vi "Find Slope and Intercept.vi"() -> ()   [LabVIEW 2020]
uses:
  Control/State - eFGV.ctl
  <vilib>/Analysis/NI_AALPro.lvlib
  <vilib>/Analysis/6fits.llb/Curve Fitting Criteria.ctl
  <vilib>/DAQmx/create/channels.llb/DAQmx Create Channel (AI-Pressure-Bridge-Table).vi
panel:
  in  "Delete index (row)":i32
  in  "Delete":bool
  out "intercept":dbl=-0.0
  out "slope":dbl=1000.0
  in  "Insert":bool
  in  "Readings":dbl[][](array[numeric])=[[0.0315564, 0.0], [0.22232425212860107, 573.0], [0.36340194940567017, 994.0], [0.7131384611129761, 2041.0], [1.0534383058547974, 3060.0], [1.3849239349365234, 4052.0], [1.7391854524612427, 5112.0], [2.0930733680725098, 6170.0], [2.4199507236480713, 7148.0], [2.762993812561035, 8174.0], [3.096597909927368, 9172.0], [3.4271647930145264, 10161.0], [3.730435609817505, 11067.0], [4.083857536315918, 12126.0], [4.432881832122803, 13172.0], [4.811169147491455, 14314.0], [5.0111083984375, 15151.0], [5.050300121307373, 16137.0], [5.08100700378418, 17097.0], [5.111919403076172, 18072.0], [5.147753715515137, 19172.0], [5.178903102874756, 20156.0], [5.262630939483643, 22859.0], [5.2826104164123535, 23500.0]]
  out "Sensor Reading (AI0)":sgl=0.63656884
  in  "Real Pressure":dbl
  in  "stop":bool
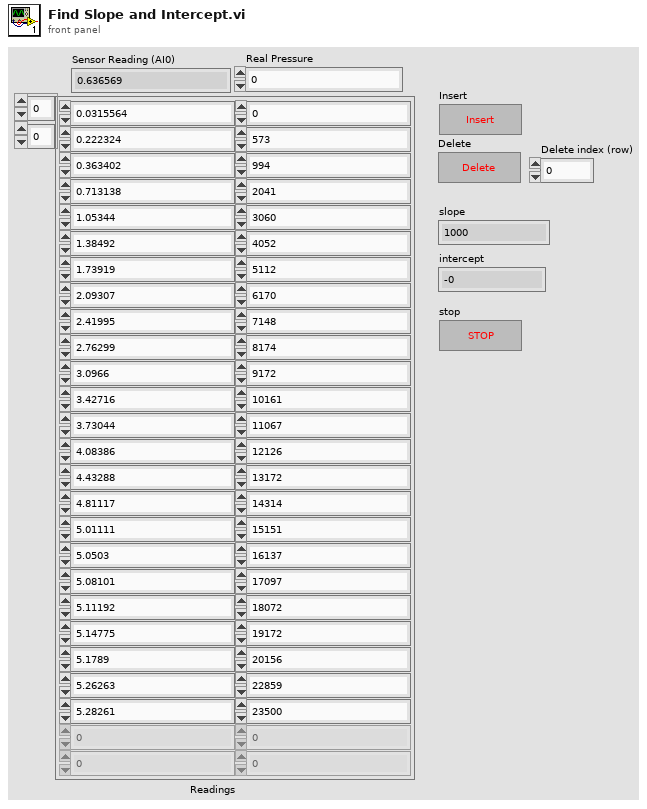
[diagram p1: front panel]
types:
  T1 = typedef "State - eFGV.ctl" = enum16{"Init", "Read", "Write", "Exit"}
  T2 = typedef "NI_AALPro.lvlib/Curve Fitting Criteria.ctl" = u16
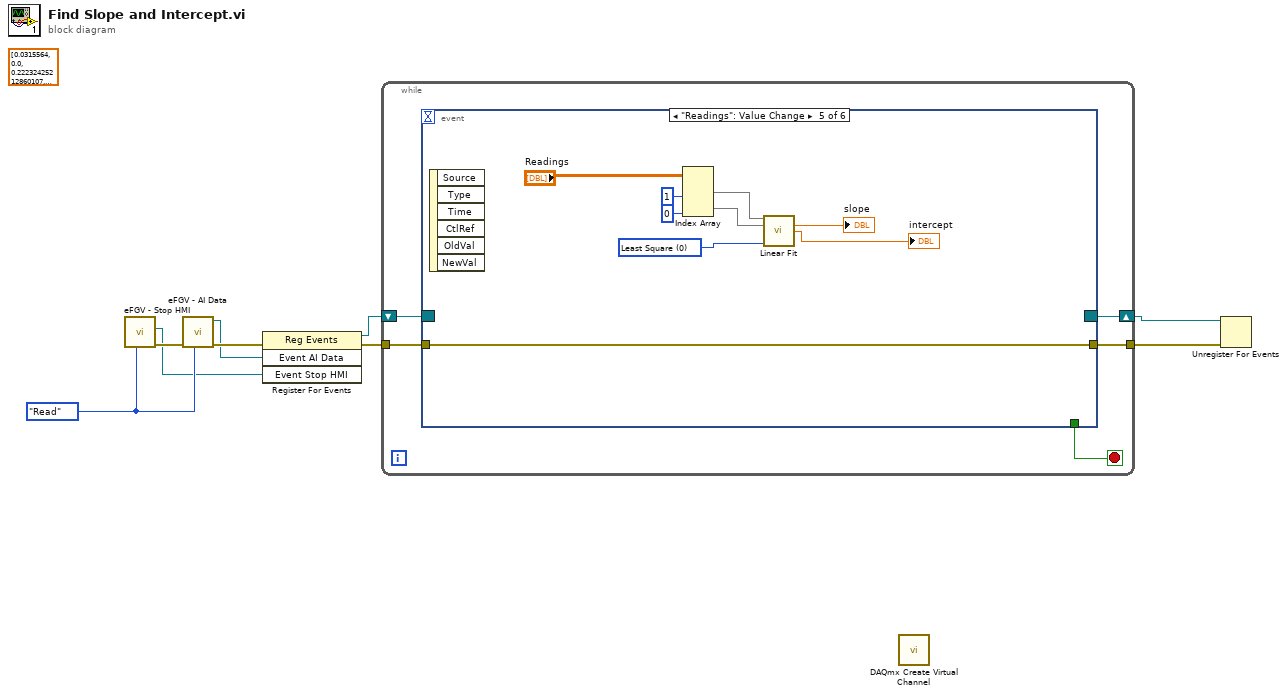
[diagram p0: block diagram]
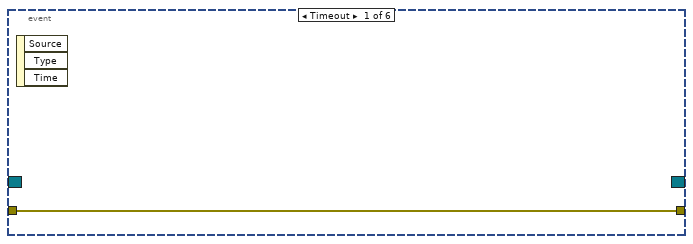
[diagram p2: hidden frame]
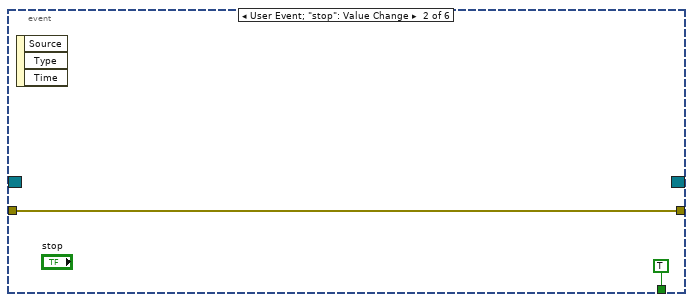
[diagram p3: hidden frame]
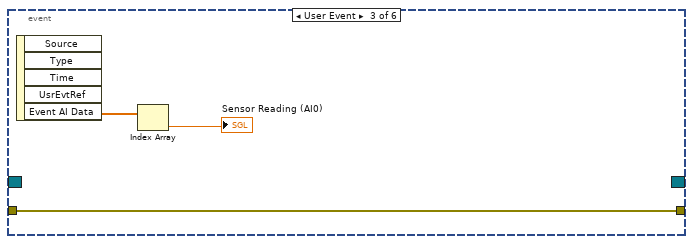
[diagram p4: hidden frame]
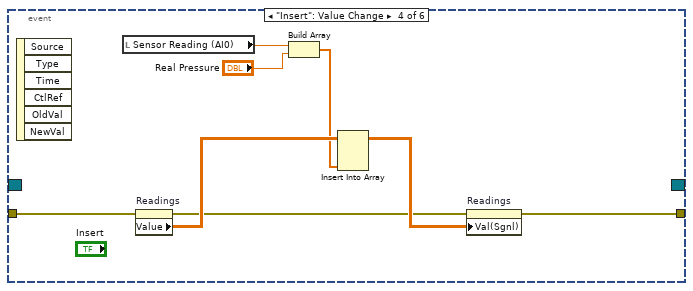
[diagram p5: hidden frame]
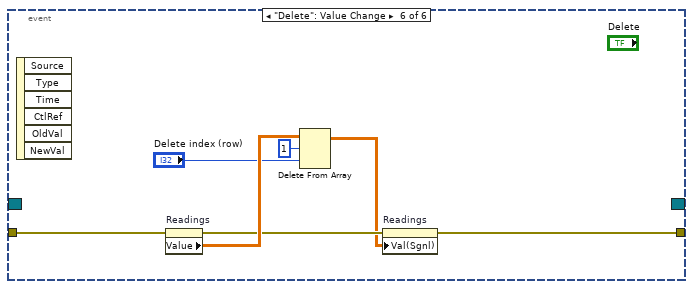
[diagram p6: hidden frame]
diagram:
  (unwired) dbl[][] [[0.0315564, 0.0], [0.22232425212860107, 573.0], [0.36340194940567017, 994.0], [0.7131384611129761, 2041.0], [1.0534383058547974, 3060.0], [1.3849239349365234, 4052.0], [1.7391854524612427, 5112.0], [2.0930733680725098, 6170.0], [2.4199507236480713, 7148.0], [2.762993812561035, 8174.0], [3.096597909927368, 9172.0], [3.4271647930145264, 10161.0], [3.730435609817505, 11067.0], [4.083857536315918, 12126.0], [4.432881832122803, 13172.0], [4.811169147491455, 14314.0], [5.0111083984375, 15151.0], [5.050300121307373, 16137.0], [5.08100700378418, 17097.0], [5.111919403076172, 18072.0], [5.147753715515137, 19172.0], [5.178903102874756, 20156.0], [5.262630939483643, 22859.0], [5.2826104164123535, 23500.0]] ("Readings")
  w4 = State_-_eFGV."Read" ("States")
  n1 = call "eFGV - Stop HMI.vi"("Action"=w4) -> ("Error Out"=w5:errorcluster, "Event Stop HMI"=w3:refnum<user-event>)  [unwired: 8 in, 1 out]
  n2 = call "eFGV - AI Data.vi"("States"=w4, "Error In"=w5) -> ("Error Out"=w9:errorcluster, "Event AI Data"=w6:refnum<user-event>)  [unwired: 8 in]
  n3 = register-events(error in=w9, w6, w3) -> (reference out=w7:refnum<event-registration>, error out=w8:errorcluster)  [unwired: 1 in]
  n4 = while {
    tunnel: w8 -> [w14]
    shift-right: [w12] -> w1
    shift-left: w7 -> [w13]
    tunnel: [w11] -> w2
    stop <- w10 stop-if-true
    n5 = event shown="[4] \"Readings\": Value Change" {
      selector: w13 -> [_ _ _ _ _ _]
      dyn-events: [_ _ _ _ _ _] -> w12
      timeout: _ -> [_ _ _ _ _ _]
      tunnel: w14 -> [w15 w17 w18 w28 w29 w44]
      tunnel: [w15 w17 w18 w25 w29 w38] -> w11
      tunnel: [_ TRUE _ _ _ _] -> w10
      event Timeout {
        n6 = event-data() -> ()  [unwired: 1 in, 3 out]
      }
      event User Event; "stop": Value Change {
        n7 = event-data() -> ()  [unwired: 1 in, 3 out]
      }
      event User Event {
        n8 = event-data() -> ("Event AI Data"=w20:sgl[])  [unwired: 1 in, 4 out]
        n9 = Index Array(array=w20) -> (element=→"Sensor Reading (AI0)":sgl)  [unwired: 1 in]
      }
      event "Insert": Value Change {
        n10 = event-data() -> ()  [unwired: 1 in, 6 out]
        n11 = local read "Sensor Reading (AI0)"() -> (w23:sgl)
        n12 = property on="Readings" class="Arr (strict)"(error in=w28) -> (error out=w24:errorcluster, "Value"=w27:dbl[][])  [unwired: 1 in, 1 out]
        n13 = Build Array(w23, "Real Pressure") -> (w21:dbl[])
        n14 = Insert Into Array(array=w27, new element=w21) -> (w26:dbl[][])  [unwired: 2 in]
        n15 = property on="Readings" class="Arr (strict)"(error in=w24, "Val(Sgnl)"=w26) -> (error out=w25:errorcluster)  [unwired: 1 in, 1 out]
      }
      event "Readings": Value Change {
        w37 = T2 0 items=["Least Square", "Least Absolute Residual", "Bisquare"] ("method")
        n16 = event-data() -> ()  [unwired: 1 in, 6 out]
        n17 = Index Array(array="Readings", index (col) #1=1 ("disabled index (col)"), index (col) #2=0 ("index (col)")) -> (element #1=w33:dbl[], element #2=w32:dbl[])  [unwired: 2 in]
        n18 = call <vilib>:"Linear Fit.vi"("Y"=w33, "X"=w32, "method"=w37) -> ("slope"=→"slope":dbl, "intercept"=→"intercept":dbl)  [unwired: 8 in, 3 out]
      }
      event "Delete": Value Change {
        n19 = event-data() -> ()  [unwired: 1 in, 6 out]
        n20 = property on="Readings" class="Arr (strict)"(error in=w44) -> (error out=w40:errorcluster, "Value"=w43:dbl[][])  [unwired: 1 in, 1 out]
        n21 = Delete From Array(array=w43, length=1, index (row)="Delete index (row)") -> (array with subset deleted=w39:dbl[][])  [unwired: 1 in, 1 out]
        n22 = property on="Readings" class="Arr (strict)"(error in=w40, "Val(Sgnl)"=w39) -> (error out=w38:errorcluster)  [unwired: 1 in, 1 out]
      }
    }
  }
  n23 = call-poly <vilib>:"DAQmx Create Virtual Channel.vi"() -> ()  [unwired: 14 in, 2 out]
  n24 = Unregister For Events(event registration refnum=w1, error in=w2) -> ()  [unwired: 1 out]
